vi "const_block.vi"(2 "Control":T3, 3 "B":T4, 4 "A":T5) -> (0 "Flags":T1, 1 "Result":T2)   [LabVIEW 2013]
panel:
  # "R1"
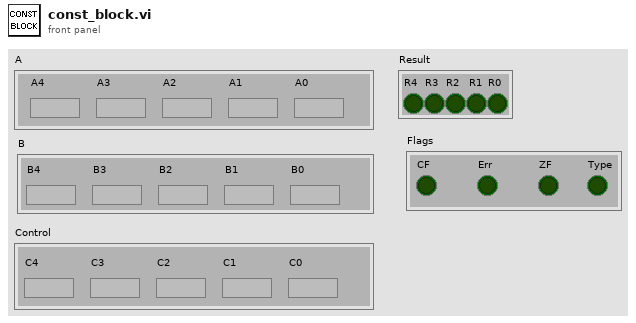
[diagram p1: front panel]
types:
  T1 = cluster{"CF":bool, "Err":bool, "ZF":bool, "Type":bool}
  T2 = cluster{"R4":bool, "R3":bool, "R2":bool, bool, "R0":bool}
  T3 = cluster{"C4":bool, "C3":bool, "C2":bool, "C1":bool, "C0":bool}
  T4 = cluster{"B4":bool, "B3":bool, "B2":bool, "B1":bool, "B0":bool}
  T5 = cluster{"A4":bool, "A3":bool, "A2":bool, "A1":bool, "A0":bool}
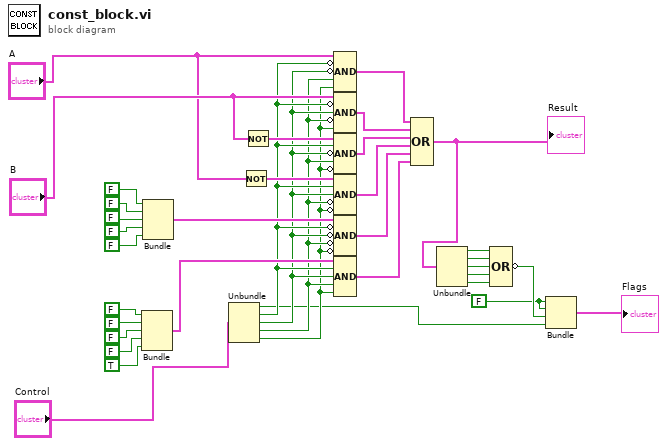
[diagram p0: block diagram]
diagram:
  w24 = FALSE
  n1 = Bundle(FALSE, FALSE, FALSE, FALSE, TRUE) -> (w7:cluster{bool, bool, bool, bool, bool})  [unwired: 1 in]
  n2 = Bundle(FALSE, FALSE, FALSE, FALSE, FALSE) -> (w6:cluster{bool, bool, bool, bool, bool})  [unwired: 1 in]
  n3 = Unbundle("Control") -> ("C4"=w1:bool, "C3"=w5:bool, "C2"=w4:bool, "C1"=w3:bool, "C0"=w2:bool)
  n4 = Not(x="A") -> (.not. x?=w20:T5)
  n5 = Not(x="B") -> (.not. x?=w21:T4)
  n6 = Compound Arithmetic op=AND("A", invert w5, invert w4, w3, w2) -> (w37:T5)
  n7 = Compound Arithmetic op=AND("B", invert w5, w4, invert w3, w2) -> (w36:T4)
  n8 = Compound Arithmetic op=AND(w21, w5, invert w4, w3, invert w2) -> (w35:T4)
  n9 = Compound Arithmetic op=AND(w20, w5, w4, invert w3, invert w2) -> (w34:T5)
  n10 = Compound Arithmetic op=AND(w6, invert w5, invert w4, invert w3, invert w2) -> (w19:cluster{bool, bool, bool, bool, bool})
  n11 = Compound Arithmetic op=AND(w7, w5, w4, w3, w2) -> (w18:cluster{bool, bool, bool, bool, bool})
  n12 = Compound Arithmetic op=OR(w37, w36, w35, w34, w19, w18) -> (w31:cluster{bool, bool, bool, bool, bool})
  "Result" <- w31
  n13 = Unbundle(w31) -> (w30:bool, w29:bool, w28:bool, w27:bool, w26:bool)
  n14 = Compound Arithmetic op=OR(w30, w29, w28, w27, w26) -> (invert w25:bool)
  n15 = Bundle(w24, w24, w25, "C4"=w1) -> (→"Flags":cluster{bool, bool, bool, "C4":bool})  [unwired: 1 in]
